vi "Save Node Image.vi"(8 "error in (no error)":errorcluster, 10 "Image Path":path, 11 "Object in":refnum<vi>) -> (0 "error out":errorcluster, 3 "Object out":refnum<vi>)   [LabVIEW 2024]
uses:
  <vilib>/Utility/miscctls.llb/LVPointTypeDef.ctl
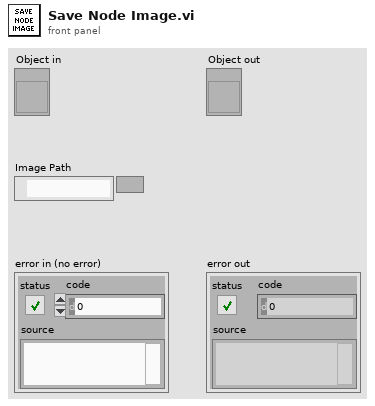
[diagram p1: front panel]
types:
  T1 = typedef "LVPointTypeDef.ctl" = cluster{"Horizontal":i16, "Vertical":i16}
  T2 = typedef "imagedata.ctl" = cluster{"image type":i32, "image depth":i32, "image":u8[], "mask":u8[], "colors":u32[], "Rectangle":cluster{"left":i16, "top":i16, "right":i16, "bottom":i16}}
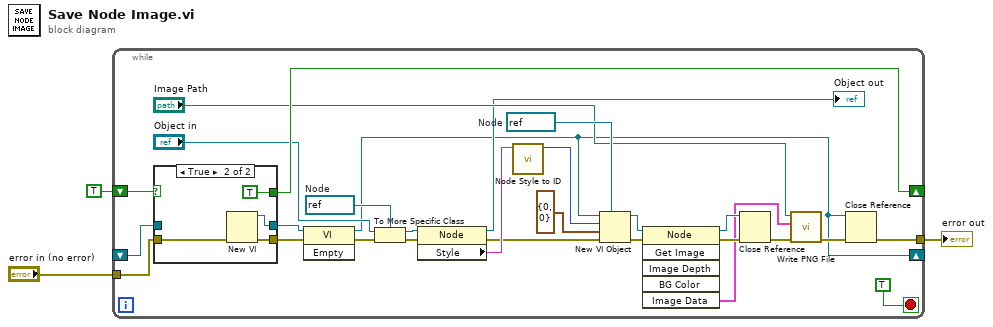
[diagram p0: block diagram]
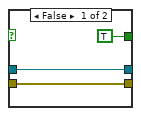
[diagram p2: hidden frame]
diagram:
  n1 = while {
    shift-right: [w29] -> _
    shift-left: TRUE -> [w30]
    shift-right: [w4] -> _
    shift-left: _ -> [w31]
    tunnel: "error in (no error)" -> [w27]
    tunnel: [w5] -> w2
    stop <- TRUE stop-if-true
    w25 = refnum<vi> refnum  # Node
    w26 = refnum<vi> refnum  # Node
    n2 = case shown="True" w30 {
      tunnel: w31 -> [w34 _]
      tunnel: [w34 w37] -> w15
      tunnel: [TRUE ("Boolean") TRUE ("Boolean")] -> w29
      tunnel: w27 -> [w32 w36]
      tunnel: [w32 w35] -> w17
      frame False {
      }
      frame True {
        n3 = New VI(8:w36) -> (0:w35:errorcluster, 3:w37:refnum<vi>)  [unwired: 6 in]
      }
    }
    n4 = invoke class="VI" method="Empty"(reference=w15, error in=w17) -> (reference out=w4:refnum<vi>, error out=w23:errorcluster)  [unwired: 1 in, 1 out]
    n5 = To More Specific Class(target class=w26, reference="Object in", error in=w23) -> (specific class reference=w22:refnum<vi>, error out=w21:errorcluster)
    n6 = property class="Node"(reference=w22, error in=w21) -> (reference out=→"Object out":refnum<vi>, error out=w19:errorcluster, "Style"=w20:string)
    n7 = call "Node Style to ID.vi"("Function Name"=w20) -> ("Function ID"=w24:i32)  [unwired: 9 in, 1 out]
    n8 = New VI Object(vi object class=w25, owner refnum=w4, style=w24, position/next to=T1 {"Horizontal"=0, "Vertical"=0} ("location"), 8:w19) -> (object refnum=w14:refnum<vi>, 0:w12:errorcluster)  [unwired: 3 in]
    n9 = invoke class="Node" method="Get Image"(reference=w14, error in=w12) -> (reference out=w13:refnum<vi>, error out=w11:errorcluster, "Image Data"=w10:T2)  [unwired: 4 in, 3 out]
    n10 = Close Reference(reference=w13, error in (no error)=w11) -> (error out=w16:errorcluster)
    n11 = call <vilib>:"Write PNG File.vi"("error in (no error)"=w16, "image data"=w10, "path to PNG file"="Image Path") -> ("error out"=w9:errorcluster)  [unwired: 7 in, 1 out]
    n12 = Close Reference(reference=w4, error in (no error)=w9) -> (error out=w5:errorcluster)
  }
  "error out" <- w2
